vi "UtilityLib.VI-Tree.vi"   [LabVIEW 2014, in "UtilityLib.lvlib"]
doc: "VI Tree, contains all VIs of UtilityLib"
uses:
  UtilityLib.lvlib
  UtilityLib.valueStatus.ctl
  UtilityLib.Operation System.ctl
  UtilityLib.helpType.ctl
types:
  T1 = typedef "UtilityLib.lvlib/UtilityLib.helpType.ctl" = enum16{"unknown", "menu", "description", "about", "special0", "special1", "special2"}
  T2 = typedef "UtilityLib.lvlib/UtilityLib.Operation System.ctl" = enum16{"unknown", "Windows", "Embedded", "RT", "Mac", "Unix", "PocketPC"}
  T3 = typedef "UtilityLib.lvlib/UtilityLib.valueStatus.ctl" = enum16{"no info available", "stand by/off", "on", "warning", "alarm/malfunction", "not implemented", "user action required", "important information", "system default", "control default", "indicator default", "button default"}
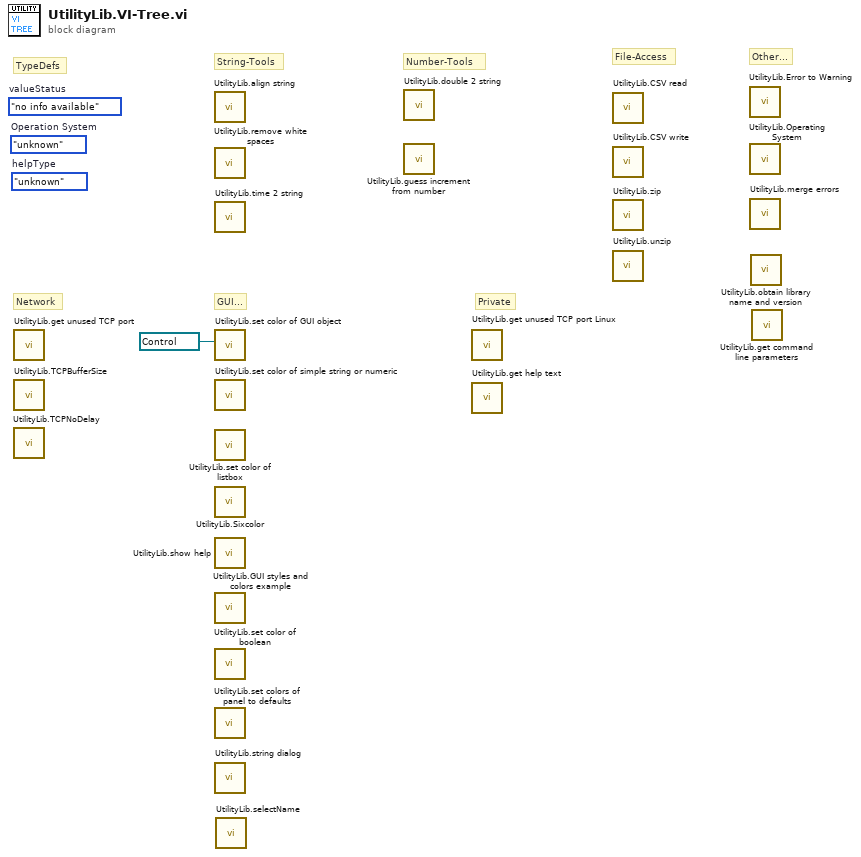
[diagram p0: block diagram]
diagram:
  (unwired) UtilityLib.helpType."unknown"  # helpType
  (unwired) UtilityLib.Operation_System."unknown"  # Operation System
  (unwired) UtilityLib.valueStatus."no info available"  # valueStatus
  # "GUI..."
  # "Network"
  # "Other..."
  # "File-Access"
  # "Number-Tools"
  # "String-Tools"
  # "Private"
  # "TypeDefs"
  n1 = call "UtilityLib.get unused TCP port.vi"() -> ()  [unwired: 18 in, 2 out]
  n2 = call "UtilityLib.TCPBufferSize.vi"() -> ()  [unwired: 10 in, 2 out]
  n3 = call "UtilityLib.TCPNoDelay.vi"() -> ()  [unwired: 10 in, 2 out]
  n4 = call "UtilityLib.align string.vi"() -> ()  [unwired: 18 in, 2 out]
  n5 = call "UtilityLib.remove white spaces.vi"() -> ()  [unwired: 15 in, 5 out]
  n6 = call "UtilityLib.time 2 string.vi"() -> ()  [unwired: 1 in, 1 out]
  n7 = call "UtilityLib.set color of GUI object.vi"("GUI object Ref"=refnum<vi> refnum) -> ()  [unwired: 18 in, 1 out]
  n8 = call "UtilityLib.set color of simple string or numeric.vi"() -> ()  [unwired: 19 in, 1 out]
  n9 = call "UtilityLib.set color of listbox.vi"() -> ()  [unwired: 19 in, 1 out]
  n10 = call "UtilityLib.Sixcolor.vi"() -> ()  [unwired: 3 in, 4 out]
  n11 = call "UtilityLib.show help.vi"() -> ()  [unwired: 1 in]
  n12 = call "UtilityLib.GUI styles and colors example.vi"() -> ()  [unwired: 1 in]
  n13 = call "UtilityLib.set color of boolean.vi"() -> ()  [unwired: 19 in, 1 out]
  n14 = call "UtilityLib.set colors of panel to defaults.vi"() -> ()  [unwired: 19 in, 1 out]
  n15 = call "UtilityLib.string dialog.vi"() -> ()  [unwired: 12 in, 4 out]
  n16 = call "UtilityLib.selectName.vi"() -> ()  [unwired: 17 in, 3 out]
  n17 = call "UtilityLib.double 2 string.vi"() -> ()  [unwired: 18 in, 2 out]
  n18 = call "UtilityLib.guess increment from number.vi"() -> ()  [unwired: 1 in, 1 out]
  n19 = call "UtilityLib.get unused TCP port Linux.vi"() -> ()  [unwired: 18 in, 2 out]
  n20 = call "UtilityLib.get help text.vi"() -> ()  [unwired: 2 in, 1 out]
  n21 = call "UtilityLib.CSV read.vi"() -> ()  [unwired: 18 in, 2 out]
  n22 = call "UtilityLib.CSV write.vi"() -> ()  [unwired: 19 in, 1 out]
  n23 = call "UtilityLib.zip.vi"() -> ()  [unwired: 17 in, 3 out]
  n24 = call "UtilityLib.unzip.vi"() -> ()  [unwired: 17 in, 3 out]
  n25 = call "UtilityLib.Error to Warning.vi"() -> ()  [unwired: 15 in, 1 out]
  n26 = call "UtilityLib.Operating System.vi"() -> ()  [unwired: 1 out]
  n27 = call "UtilityLib.merge errors.vi"() -> ()  [unwired: 2 in, 1 out]
  n28 = call "UtilityLib.obtain library name and version.vi"() -> ()  [unwired: 1 in, 1 out]
  n29 = call "UtilityLib.get command line parameters.vi"() -> ()  [unwired: 9 in, 3 out]
